vi "Create.vi"(10 "Value":dbl) -> (3 "DoubleValue":refnum<class "DoubleValue.lvclass">)   [LabVIEW 2020, in "Futures-Examples.lvlib" / "DoubleValue.lvclass"]
uses:
  DoubleValue.lvclass
  DoubleValue.lvclass/DoubleValue.ctl
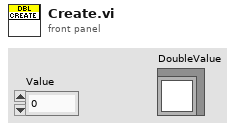
[diagram p1: front panel]
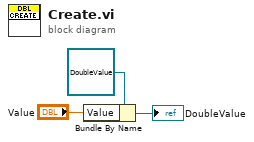
[diagram p0: block diagram]
diagram:
  n1 = Bundle By Name(cluster=refnum<class "DoubleValue.lvclass"> refnum ("DoubleValue"), "Value"="Value") -> (→"DoubleValue":refnum<class "DoubleValue.lvclass">)
